vi "DBC Get Signal Value Str.vi"(7 "pValueStr":string, 9 "pSignalName":string, 10 "pMsgName":string, 11 "DBCHandle":u64) -> (1 "pSignalName out":string, 2 "pMsgName out":string, 3 "function return":i32, 5 "pValueStr out":string)   [LabVIEW 2010, in "dbc_parser.lvlib"]
doc: "int WINAPI DBC_GetSignalValueStr(long long DBCHandle, char* pMsgName, char* pSignalName, char* pValueStr);"
uses:
  dbc_parser.lvlib
  USB2XXX/trunk/USB2XXX/USB2XXX/vs2019/Release/USB2XXX.dll
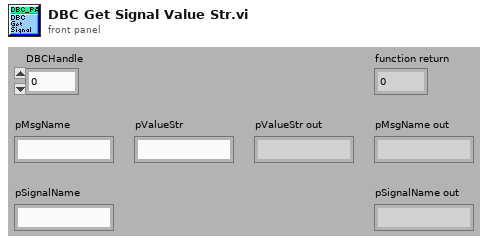
[diagram p1: front panel]
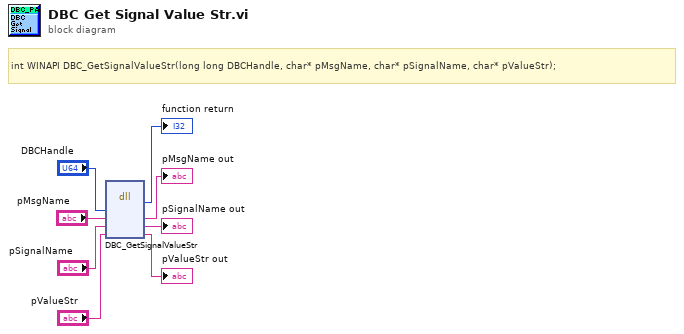
[diagram p0: block diagram]
diagram:
  # "int WINAPI DBC_GetSignalValueStr(long long DBCHandle, char* pMsgName, char* pSignalName, char* pValueStr);"
  n1 = dll-call lib="E:/Projects/USB2XXX/trunk/USB2XXX/USB2XXX/vs2019/Release/USB2XXX.*" fn="DBC_GetSignalValueStr"("DBCHandle"="DBCHandle", "pMsgName"="pMsgName", "pSignalName"="pSignalName", "pValueStr"="pValueStr") -> (→"function return":i32, "pMsgName"=→"pMsgName out":string, "pSignalName"=→"pSignalName out":string, "pValueStr"=→"pValueStr out":string)  [unwired: 4 in, 2 out]
